vi "LEP_RV_OnProfile.vi"(8 "error in (no error)":errorcluster) -> (0 "error out":errorcluster)   [LabVIEW 2011]
doc: "Download and execute built VxWorks downloadable module and attach the LabVIEW Embedded debuger."
uses:
  LEP_RV_Commands.ctl
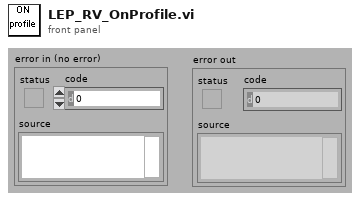
[diagram p1: front panel]
types:
  T1 = typedef "LEP_RV_Commands.ctl" = enum16{"Build", "Rebuild", "Run", "Debug", "Profile"}
  T2 = typedef "LEP_RV_Config.ctl" = cluster{"Enable debugging":bool, "Debug Options":u16, "Use stack variables":bool, "Generate serial only":bool, "Generate guard code":bool, "Generate Integer Only":bool, "Generate C Function Calls":bool, "ExpressionFolding":bool, "Constant Allocation":u16, "Constant Deallocation":u16, "Build Specification ID":string, "Preprocessor symbols (define)":string, "Compiler Flags":string, "Linker Flags":string, "Mode":u16, "Optimization":u16, "Optimize for time":bool, "Enable cross-module optimization":bool, "Include paths":path[], "Optimize heap size":bool, "Use MicroLib":bool, "Debug Mode":u16, "Enable profile information":bool, "Host name":string, "Use DHCP":bool, "IP address":string, "Subnet mask":string, "Gateway":string, "Primary DNS":string, "Secondary DNS":string, "MAC in target memory":bool, "MAC address":string, "Console output":u16, "Target serial port":u16}
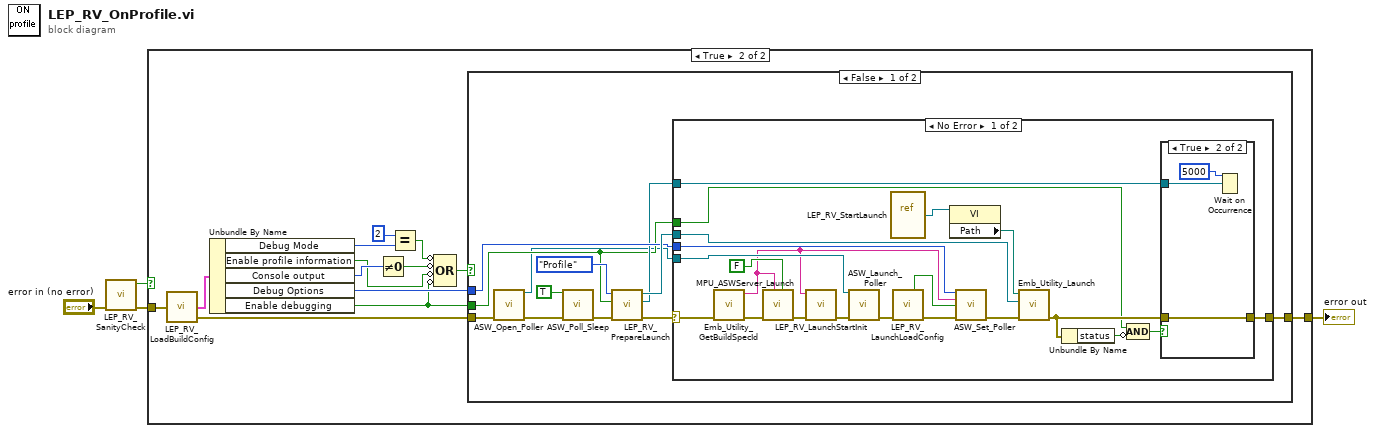
[diagram p0: block diagram]
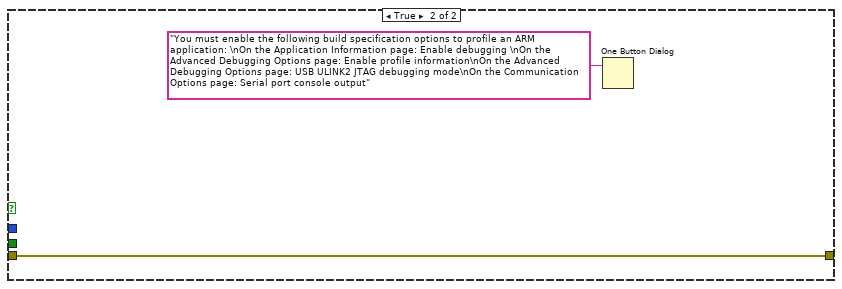
[diagram p5: hidden frame]
diagram:
  n1 = call "LEP_RV_SanityCheck.vi"("error in (no error)"="error in (no error)") -> ("error out"=w2:errorcluster, "ok"=w1:bool)  [unwired: 1 in, 8 out]
  n2 = case shown="True" w1 {
    tunnel: [w5 w16] -> w3
    tunnel: w2 -> [w5 w15]
    frame False {
    }
    frame True {
      n3 = call "LEP_RV_LoadBuildConfig.vi"("error in (no error)"=w15) -> ("Config"=w18:T2, "error out"=w14:errorcluster)  [unwired: 1 out]
      n4 = Unbundle By Name(w18) -> ("Debug Mode"=w9:u16, "Enable profile information"=w7:bool, "Console output"=w8:u16, "Debug Options"=w17:u16, "Enable debugging"=w6:bool)
      n5 = Not Equal To 0?(x=w8) -> (x != 0?=w11:bool)
      n6 = Equal?(x=u16 2, y=w9) -> (x = y?=w12:bool)
      n7 = Compound Arithmetic op=OR(invert w12, invert w11, invert w7, invert w6) -> (w10:bool)
      n8 = case shown="False" w10 {
        tunnel: w17 -> [w28 _]
        tunnel: [w20 w58] -> w16
        tunnel: w6 -> [w25 _]
        tunnel: w14 -> [w19 w58]
        frame False {
          n9 = call <vilib>:"ASW_Open_Poller.vi"("error in (no error)"=w19) -> ("vi reference"=w22:refnum<vi>, "error out"=w24:errorcluster)  [unwired: 13 in]
          n10 = call <vilib>:"ASW_Poll_Sleep.vi"("Sleep"=TRUE, "error in (no error)"=w24) -> ("error out"=w23:errorcluster)  [unwired: 13 in]
          n11 = call "LEP_RV_PrepareLaunch.vi"("error in (no error)"=w23, "Enable debugging"=w25, "Commands"=LEP_RV_Commands."Profile") -> ("error out"=w30:errorcluster, "debug occurrence"=w27:refnum<k4>, "output cluster"=w29:refnum<vi>)  [unwired: 6 in]
          n12 = case shown="No Error" w30 {
            selector: w30 -> [w48 w56]
            tunnel: [w43 w56] -> w20
            tunnel: w29 -> [w47 _]
            tunnel: w28 -> [w44 _]
            tunnel: w27 -> [w42 _]
            tunnel: w25 -> [w35 _]
            tunnel: w22 -> [w41 _]
            frame No Error {
              n13 = call <vilib>:"Emb_Utility_GetBuildSpecId.vi"("error in (no error)"=w48) -> ("error out"=w49:errorcluster, "buildSpec ID"=w38:string)  [unwired: 7 out]
              n14 = call <vilib>:"MPU_ASWServer_Launch.vi"("initialize (T)"=FALSE, "buildSpec ID"=w38, "error in"=w49) -> ("error out"=w40:errorcluster)  [unwired: 8 out]
              n15 = call "LEP_RV_LaunchStartInit.vi"("error in (no error)"=w40, "buildSpec ID"=w38) -> ("error out"=w39:errorcluster)  [unwired: 9 in]
              n16 = call <vilib>:"ASW_Launch_Poller.vi"("reference"=w41, "error in (no error)"=w39) -> ("error out"=w33:errorcluster)  [unwired: 13 in]
              n17 = vi-ref "LEP_RV_StartLaunch.vi"() -> (w51:refnum<vi>)
              n18 = call "LEP_RV_LaunchLoadConfig.vi"("error in (no error)"=w33) -> ("Connect to a network compile server"=w31:bool, "error out"=w32:errorcluster)  [unwired: 7 in, 6 out]
              n19 = property class="VI"(reference=w51) -> ("Path"=w50:path)  [unwired: 1 in, 2 out]
              n20 = call <vilib>:"ASW_Set_Poller.vi"("Debug Options"=w44, "buildSpec ID"=w38, "Connect to a network compile server"=w31, "error in (no error)"=w32) -> ("error out"=w45:errorcluster)  [unwired: 11 in]
              n21 = call <vilib>:"Emb_Utility_Launch.vi"("error in"=w45, "parameter cluster"=w47, "vi path"=w50) -> ("error out"=w37:errorcluster)  [unwired: 6 out]
              n22 = Unbundle By Name(w37) -> ("status"=w36:bool)
              n23 = Compound Arithmetic op=AND(w35, invert w36) -> (w34:bool)
              n24 = case shown="True" w34 {
                tunnel: w37 -> [w52 w54]
                tunnel: [w52 w54] -> w43
                tunnel: w42 -> [_ w53]
                frame False {
                }
                frame True {
                  n25 = Wait on Occurrence(2:w53, 3:5000 ("ms timeout (-1)")) -> ()  [unwired: 1 in, 1 out]
                }
              }
            }
            frame Error {
            }
          }
        }
        frame True {
          n26 = One Button Dialog(message="You must enable the following build specification options to profile an ARM application: \nOn the Application Information page: Enable debugging \nOn the Advanced Debugging Options page: Enable profile information\nOn the Advanced Debugging Options page: USB ULINK2 JTAG debugging mode\nOn the Communication Options page: Serial port console output") -> ()  [unwired: 2 out]
        }
      }
    }
  }
  "error out" <- w3
